vi "deleteEmptyDevices.vi"(8 "error in (no error)":errorcluster, 11 "DeviceArray in":refnum<class "DeviceArray.lvclass">) -> (0 "error out":errorcluster, 3 "DeviceArray out":refnum<class "DeviceArray.lvclass">)   [LabVIEW 2011, in "Tools.lvlib" / "DatabaseHelpers.lvlib" / "DeviceArray.lvclass"]
uses:
  DeviceArray.lvclass
  device/device.lvclass
  DeviceArray.lvclass/DeviceArray.ctl
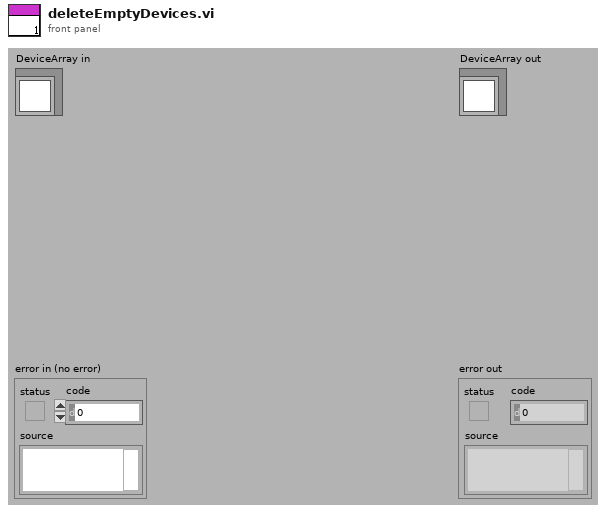
[diagram p1: front panel]
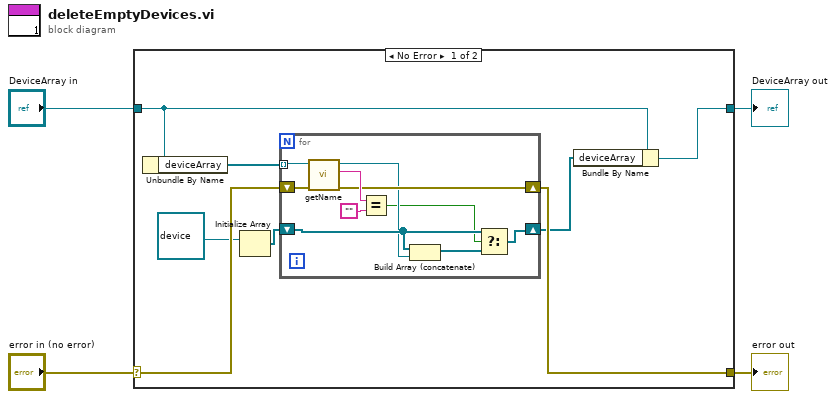
[diagram p0: block diagram]
diagram:
  n1 = case shown="No Error" "error in (no error)" {
    selector: "error in (no error)" -> [w12 w24]
    tunnel: [w8 w24] -> w3
    tunnel: [w5 w23] -> w1
    tunnel: "DeviceArray in" -> [w6 w23]
    frame No Error {
      n2 = Unbundle By Name(w6) -> ("deviceArray"=w10:refnum<class "device.lvclass">[])
      n3 = Initialize Array(refnum<class "device.lvclass"> refnum ("Tools.lvlib:DatabaseHelpers.lvlib:device.lvclass")) -> (w11:refnum<class "device.lvclass">[])  [unwired: 1 in]
      n4 = for {
        tunnel: w10 -> [w22] mode=indexing
        shift-right: [w18] -> w8
        shift-left: w12 -> [w21]
        shift-right: [w13] -> w7
        shift-left: w11 -> [w17]
        n5 = call "getName.vi"("error in (no error)"=w21, "device.lvclass in"=w22) -> ("error out"=w18:errorcluster, "name"=w19:string, "device.lvclass out"=w16:refnum<class "device.lvclass">)  [unwired: 7 in]
        n6 = Equal?(x=w19, y="") -> (x = y?=w15:bool)
        n7 = Build Array (concatenate)(w17, w16) -> (w14:refnum<class "device.lvclass">[])
        n8 = Select(t=w17, s=w15, f=w14) -> (s? t:f=w13:refnum<class "device.lvclass">[])
      }
      n9 = Bundle By Name(cluster=w6, "deviceArray"=w7) -> (w5:refnum<class "DeviceArray.lvclass">)
    }
    frame Error {
    }
  }
  "error out" <- w3
  "DeviceArray out" <- w1
